vi "Parse Basic String.vi"(8 "error in (no error)":errorcluster, 10 "start at":i32, 11 "TOML String":string) -> (0 "error out":errorcluster, 2 "offset past match":i32, 3 "String":string)   [LabVIEW 2019, in "BlueTOMLSerializer.lvlib"]
uses:
  BlueTOMLSerializer.lvlib
  <vilib>/regexp/Match Regular Expression.xnode
panel:
  out "before match":string
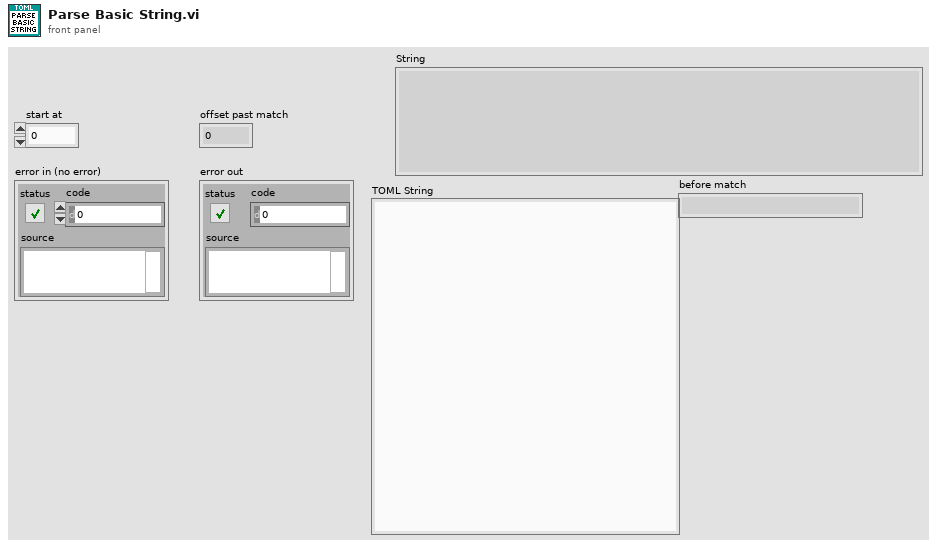
[diagram p1: front panel]
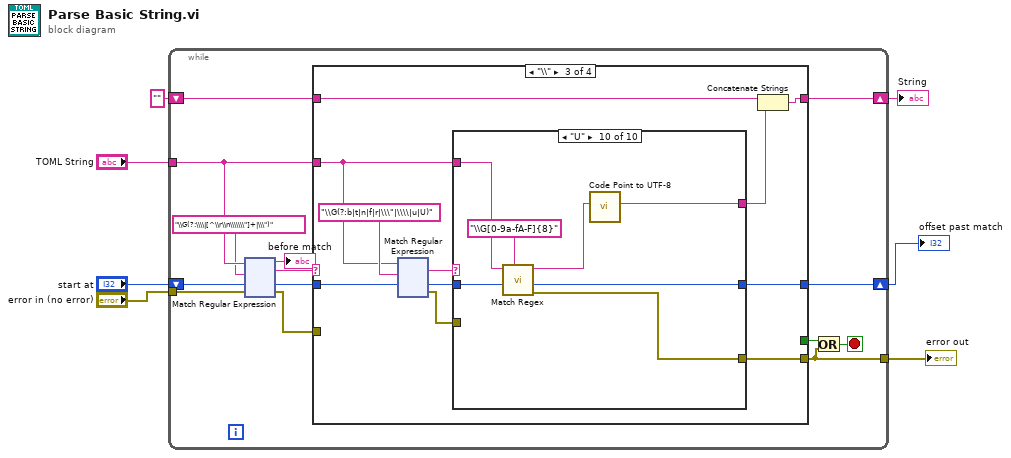
[diagram p0: block diagram]
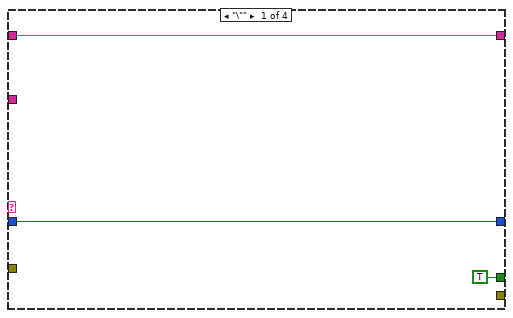
[diagram p2: hidden frame]
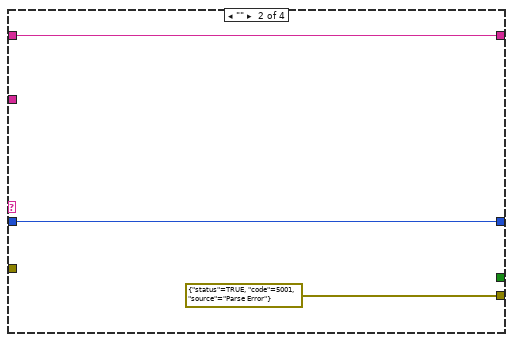
[diagram p3: hidden frame]
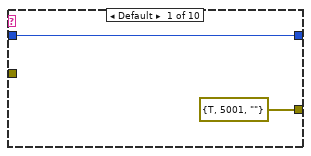
[diagram p4: hidden frame]
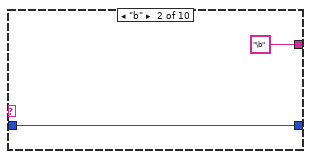
[diagram p5: hidden frame]
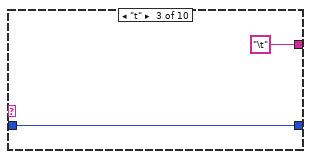
[diagram p6: hidden frame]
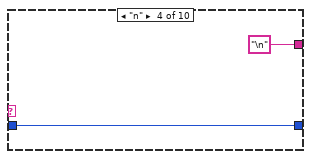
[diagram p7: hidden frame]
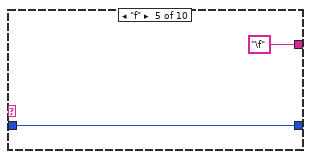
[diagram p8: hidden frame]
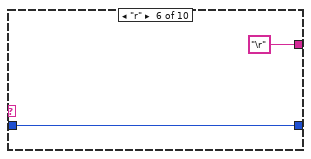
[diagram p9: hidden frame]
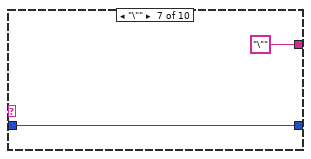
[diagram p10: hidden frame]
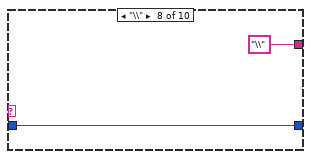
[diagram p11: hidden frame]
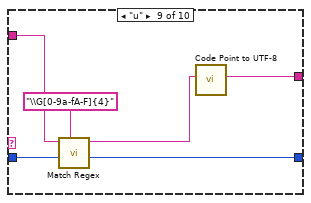
[diagram p12: hidden frame]
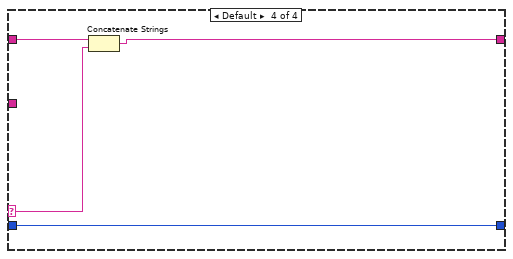
[diagram p13: hidden frame]
diagram:
  n1 = while {
    tunnel: "error in (no error)" -> [w21]
    tunnel: "TOML String" -> [w14]
    shift-right: [w19] -> w1
    shift-left: "start at" -> [w20]
    shift-right: [w17] -> w2
    shift-left: "" -> [w16]
    tunnel: [w12] -> w3
    stop <- w13 stop-if-true
    n2 = xnode "Match Regular Expression"("input string"=w14, "regular expression"="\\G(?:\\\\|[^\\r\\n\\\\\\\"]+|\\\")", "offset (0)"=w20, "error in"=w21) -> ("before match"=→"before match":string, "whole match"=w11:string, "offset past match"=w18:i32, "error out"=w9:errorcluster)  [unwired: 2 in, 1 out]
    n3 = case shown="\"\\\\\"" w11 {
      selector: w11 -> [_ _ _ w184]
      tunnel: [w23 w26 w34 w185] -> w19
      tunnel: w18 -> [w23 w26 w37 w185]
      tunnel: [w24 w27 w32 w182] -> w17
      tunnel: w16 -> [w24 w27 w38 w183]
      tunnel: [TRUE _ _ _] -> w15
      tunnel: w14 -> [_ _ w30 _]
      tunnel: [_ errorcluster {"status"=TRUE, "code"=5001, "source"="Parse Error"} ("error constant") w35 _] -> w12
      tunnel: w9 -> [_ _ _ _]
      frame "\"" {
      }
      frame "" {
      }
      frame "\\" {
        n4 = xnode "Match Regular Expression"("input string"=w30, "regular expression"="\\G(?:b|t|n|f|r|\\\"|\\\\|u|U)", "offset (0)"=w37) -> ("whole match"=w29:string, "offset past match"=w33:i32, "error out"=w28:errorcluster)  [unwired: 3 in, 2 out]
        n5 = case shown="\"U\"" w29 {
          tunnel: [errorcluster {"status"=TRUE, "code"=5001, "source"=""} ("error constant") _ _ _ _ _ _ _ _ w63] -> w35
          tunnel: [w39 w41 w43 w45 w47 w49 w51 w53 w57 w64] -> w34
          tunnel: w33 -> [w39 w41 w43 w45 w47 w49 w51 w53 w58 w65]
          tunnel: [_ "\b" ("regular expression") "\t" ("regular expression") "\n" ("regular expression") "\f" ("regular expression") "\r" ("regular expression") "\"" ("regular expression") "\\" ("regular expression") w55 w61] -> w31
          tunnel: w30 -> [_ _ _ _ _ _ _ _ w59 w66]
          tunnel: w28 -> [_ _ _ _ _ _ _ _ _ _]
          frame Default {
          }
          frame "b" {
          }
          frame "t" {
          }
          frame "n" {
          }
          frame "f" {
          }
          frame "r" {
          }
          frame "\"" {
          }
          frame "\\" {
          }
          frame "u" {
            n6 = call "Match Regex.vi"("regular expression"="\\G[0-9a-fA-F]{4}", "offset"=w58, "String"=w59) -> ("offset past match"=w57:i32, "whole match"=w56:string)  [unwired: 5 in, 2 out]
            n7 = call "Code Point to UTF-8.vi"("Code Point"=w56) -> ("UTF-8"=w55:string)  [unwired: 10 in]
          }
          frame "U" {
            n8 = call "Match Regex.vi"("regular expression"="\\G[0-9a-fA-F]{8}", "offset"=w65, "String"=w66) -> ("error out"=w63:errorcluster, "offset past match"=w64:i32, "whole match"=w62:string)  [unwired: 5 in, 1 out]
            n9 = call "Code Point to UTF-8.vi"("Code Point"=w62) -> ("UTF-8"=w61:string)  [unwired: 10 in]
          }
        }
        n10 = Concatenate Strings(w38, w31) -> (w32:string)
      }
      frame Default {
        n11 = Concatenate Strings(w183, w184) -> (w182:string)
      }
    }
    n12 = Or(x=w15, y=w12) -> (x .or. y?=w13:bool)
  }
  "error out" <- w3
  "offset past match" <- w1
  "String" <- w2
